vi "Stop DC meter.vi"(8 "error in (no error)":errorcluster, 11 "DC meter":T1={"DC meter type"=enum."H/A/K 3458", "DC meter VISA"="", "NPLC"=10.0, "status ref"=refnum}) -> (0 "error out":errorcluster, 3 "DC meter out":T1={"DC meter type"=enum."H/A/K 3458", "DC meter VISA"="", "NPLC"=10.0, "status ref"=refnum})   [LabVIEW 2020]
doc: "Close communication with DC meter."
uses:
  Type definitions/DC meter.ctl
  Type definitions/DC meter type.ctl
  external libraries/Fluke 8508/Fluke 8508.lvlib
  external libraries/3458A Basic Driver/3458A Basic Driver.lvlib
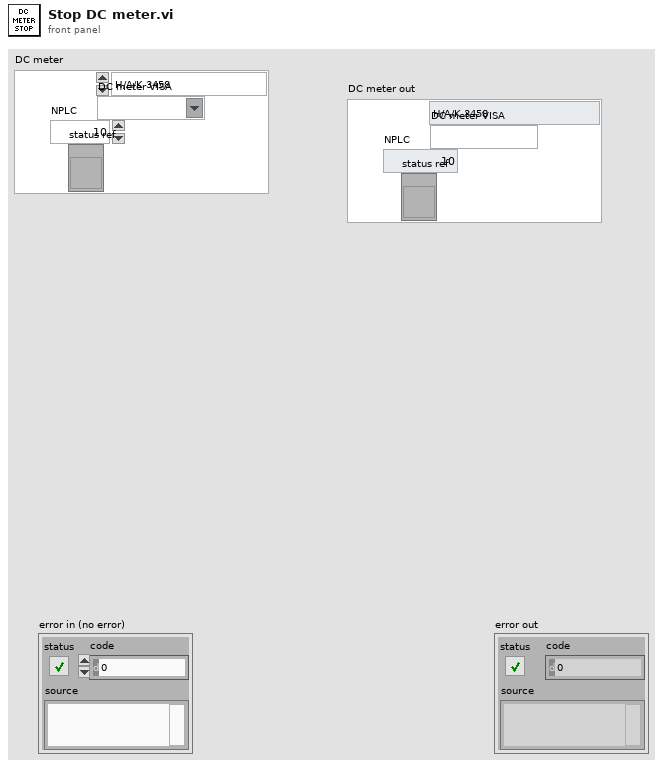
[diagram p1: front panel]
types:
  T1 = typedef "DC meter.ctl" = cluster{"DC meter type":T2, "DC meter VISA":refnum<visa-resource-name>, "NPLC":dbl, "status ref":refnum<vi>}
  T2 = typedef "DC meter type.ctl" = enum16{"H/A/K 3458", "Fluke 8508A", "dummy", "Keithley 2182"}
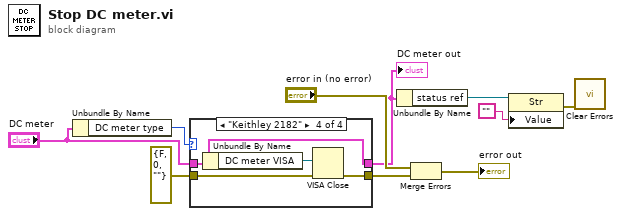
[diagram p0: block diagram]
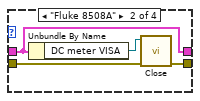
[diagram p3: hidden frame]
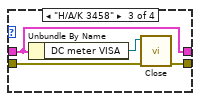
[diagram p4: hidden frame]
diagram:
  n1 = Unbundle By Name("DC meter") -> ("DC meter type"=w10:T2)
  n2 = case shown="\"Keithley 2182\"" w10 {
    tunnel: errorcluster {"status"=FALSE, "code"=0, "source"=""} ("error in (no error)") -> [w12 w14 w20 w23]
    tunnel: [w12 w13 w19 w22] -> w5
    tunnel: "DC meter" -> [w11 w16 w17 w21]
    tunnel: [w11 w16 w17 w21] -> w1
    frame "dummy" {
    }
    frame "Fluke 8508A" {
      n3 = Unbundle By Name(w16) -> ("DC meter VISA"=w15:refnum<visa-resource-name>)
      n4 = call "Close.vi"("error in (no error)"=w14, "VISA resource name"=w15) -> ("error out"=w13:errorcluster)  [unwired: 9 in]
    }
    frame "H/A/K 3458" {
      n5 = Unbundle By Name(w17) -> ("DC meter VISA"=w18:refnum<visa-resource-name>)
      n6 = call "Close.vi"("error in (no error)"=w20, "VISA resource name"=w18) -> ("error out"=w19:errorcluster)  [unwired: 9 in]
    }
    frame "Keithley 2182" {
      n7 = Unbundle By Name(w21) -> ("DC meter VISA"=w24:refnum<visa-resource-name>)
      n8 = VISA Close(VISA resource name=w24, error in (no error)=w23) -> (error out=w22:errorcluster)
    }
  }
  "DC meter out" <- w1
  n9 = Unbundle By Name(w1) -> ("status ref"=w2:refnum<vi>)
  n10 = Merge Errors("error in (no error)", w5) -> (→"error out":errorcluster)
  n11 = property class="Str"(reference=w2, "Value"="") -> (error out=w8:errorcluster)  [unwired: 1 in, 1 out]
  n12 = call <vilib>:"Clear Errors.vi"("error in (no error)"=w8) -> ()  [unwired: 5 in, 2 out]
